vi "RT_Config_sbRIO.vi"() -> (0 "error out":errorcluster, 3 "FPGA VI  Out":refnum<k20>)   [LabVIEW 2017]
uses:
  <vilib>/LabVIEW Targets/FPGA/cRIO/shared/nicrio_ModuleControls/nicrio_cRIO-9871_BaudRateEnum.ctl
  <vilib>/FPGAPlugInAG/sbRIO-9627/niLvFpga_Open_sbRIO-9627.vi
  <vilib>/rvi/interface/common/dynamic/niFpgaDynamicAddResources.vi
  <vilib>/FPGAPlugInAG/Dynamic/niLvFpga_Reset_Dynamic.vi
  <vilib>/Utility/error.llb/Error Cluster From Error Code.vi
  <vilib>/rvi/errors/niLvFpgaAdjustHostInterfaceError.vi
  <vilib>/FPGAPlugInAG/Dynamic/niLvFpga_Run_Dynamic.vi
  <vilib>/RVI Host/nirviSupport.llb/nirviErrorClusterFromErrorCode.vi
  <vilib>/rvi/interface/nirviOpenFPGA/nirviOpenFPGA.xnode
  FPGA Bitfiles/RSProject1_FPGATarget_FPGAsbFOG_nqNeV5r0bh8.lvbitx
  <vilib>/rvi/interface/nirviMethod/nirviMethod.xnode
  <vilib>/rvi/interface/nirviReadWriteControl/nirviReadWriteControl.xnode
  NiFpgaLv.dll
  <vilib>/rvi/interface/Simulation/niFpgaSimulationCallBeginRW.vi
  <vilib>/FPGAPlugInAG/Dynamic/niLvFpga_StartFifo_Dynamic.vi
  <vilib>/rvi/errors/niLvFpgaMergeErrorWithErrorCode.vi
  <vilib>/FPGAPlugInAG/Dynamic/niLvFpga_AcknowledgeIrq_Dynamic.vi
  <vilib>/rvi/interface/nirviMethod/StockFPGA_InlinedMethodWaitForSingleIRQ.vi
  <vilib>/FPGAPlugInAG/Dynamic/niLvFpga_WaitOnIrq_Dynamic.vi
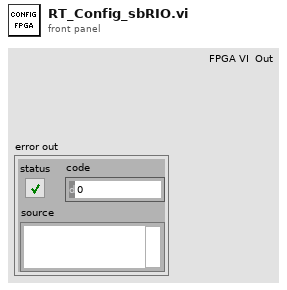
[diagram p1: front panel]
types:
  T1 = typedef "nicrio_cRIO-9871_BaudRateEnum.ctl" = enum16{"75 bps", "110 bps", "134 bps", "150 bps", "300 bps", "600 bps", "1200 bps", "1800 bps", "2400 bps", "4800 bps", "7200 bps", "9600 bps", "14.4 kbps", "19.2 kbps", "28.8 kbps", "38.4 kbps", "57.6 kbps", "115.2 kbps", "230.4 kbps", "460.8 kbps", "921.6 kbps"}
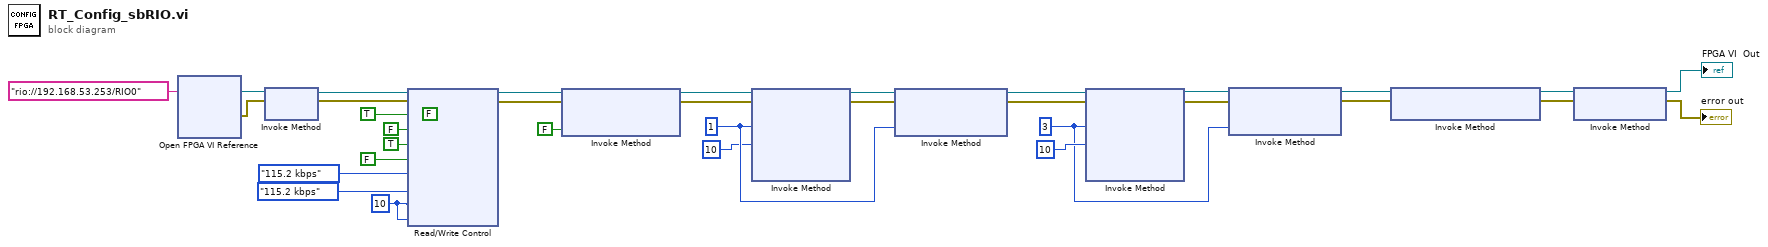
[diagram p0: block diagram]
diagram:
  w8 = 1 ("IRQ Number(s)")
  w15 = 3 ("IRQ Number(s)")
  w33 = 10 ("Timeout_FR 1")
  (unwired) FALSE ("Port1?")
  n1 = xnode "Open FPGA VI Reference"("resource name"=tag "rio://192.168.53.253/RIO0") -> ("FPGA VI Reference Out"=w21:refnum<k20>, "error out"=w22:errorcluster)  [unwired: 1 in]
  n2 = xnode "Invoke Method"("FPGA VI Reference In"=w21, "error in"=w22) -> ("FPGA VI Reference Out"=w27:refnum<k20>, "error out"=w28:errorcluster)
  n3 = xnode "Read/Write Control"("FPGA VI Reference In"=w27, "error in"=w28, "Port1?"=TRUE, "Port4?"=FALSE, "Port3?"=TRUE, "Port2?"=FALSE, "Baud Rate_P1"=nicrio_cRIO-9871_BaudRateEnum."115.2 kbps", "Baud Rate_P3"=nicrio_cRIO-9871_BaudRateEnum."115.2 kbps", "Timeout_FR 1"=w33, "Timeout_FR 2"=w33) -> ("FPGA VI Reference Out"=w25:refnum<k20>, "error out"=w26:errorcluster)
  n4 = xnode "Invoke Method"("FPGA VI Reference In"=w25, "error in"=w26, "Wait Until Done (F)"=FALSE) -> ("FPGA VI Reference Out"=w6:refnum<k20>, "error out"=w5:errorcluster)
  n5 = xnode "Invoke Method"("FPGA VI Reference In"=w6, "error in"=w5, "IRQ Number(s)"=w8, "Timeout (ms)"=10) -> ("FPGA VI Reference Out"=w4:refnum<k20>, "error out"=w3:errorcluster)  [unwired: 2 out]
  n6 = xnode "Invoke Method"("FPGA VI Reference In"=w4, "error in"=w3, "IRQ Number(s)"=w8) -> ("FPGA VI Reference Out"=w2:refnum<k20>, "error out"=w1:errorcluster)
  n7 = xnode "Invoke Method"("FPGA VI Reference In"=w2, "error in"=w1, "IRQ Number(s)"=w15, "Timeout (ms)"=10) -> ("FPGA VI Reference Out"=w14:refnum<k20>, "error out"=w13:errorcluster)  [unwired: 2 out]
  n8 = xnode "Invoke Method"("FPGA VI Reference In"=w14, "error in"=w13, "IRQ Number(s)"=w15) -> ("FPGA VI Reference Out"=w17:refnum<k20>, "error out"=w18:errorcluster)
  n9 = xnode "Invoke Method"("FPGA VI Reference In"=w17, "error in"=w18) -> ("FPGA VI Reference Out"=w12:refnum<k20>, "error out"=w11:errorcluster)
  n10 = xnode "Invoke Method"("FPGA VI Reference In"=w12, "error in"=w11) -> ("FPGA VI Reference Out"=→"FPGA VI  Out":refnum<k20>, "error out"=→"error out":errorcluster)
